vi "Recursive Delete of Registry Key.vi"(8 "error in (no error)":errorcluster, 11 "Path of Key to Delete":string) -> (0 "error out":errorcluster)   [LabVIEW 2011]
uses:
  <vilib>/registry/registry.llb/Registry refnum.ctl
  <vilib>/registry/registry.llb/Registry RtKey.ctl
  <vilib>/registry/registry.llb/Registry SAM.ctl
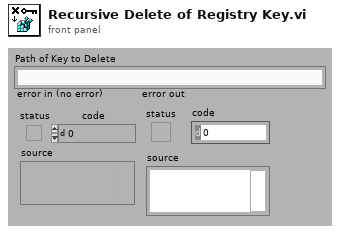
[diagram p1: front panel]
types:
  T1 = typedef "Registry SAM.ctl" = enum32{"KEY_QUERY_VALUE", "KEY_SET_VALUE", "KEY_CREATE_SUB_KEY", "KEY_ENUMERATE_SUB_KEYS", "KEY_NOTIFY", "KEY_CREATE_LINK", "KEY_READ", "KEY_WRITE", "KEY_ALL_ACCESS", "KEY_READ | KEY_WRITE"}
  T2 = typedef "Registry RtKey.ctl" = enum32{"HKEY_CLASSES_ROOT", "HKEY_CURRENT_USER", "HKEY_LOCAL_MACHINE", "HKEY_USERS", "HKEY_PERFORMANCE_DATA", "HKEY_CURRENT_CONFIG", "HKEY_DYN_DATA"}
  T3 = typedef "Registry refnum.ctl" = refnum<k1>
  T4 = cluster{"numSubKeys":i32, "maxSubKeyLen":i32, "maxSubKeyClassLen":i32}
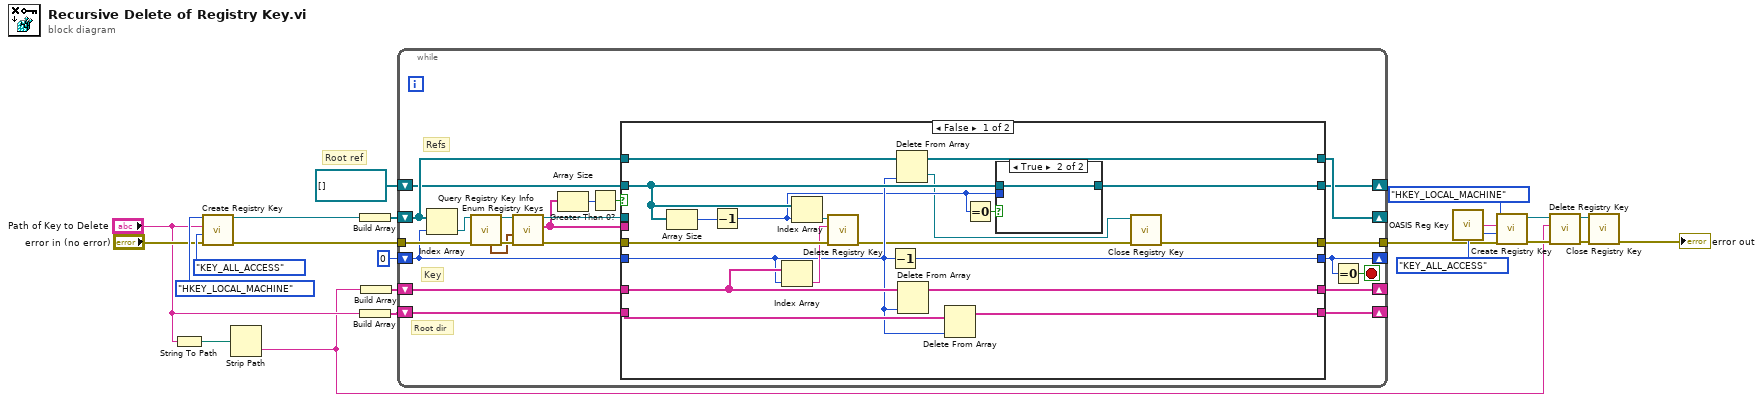
[diagram p0: block diagram]
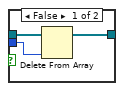
[diagram p2: hidden frame]
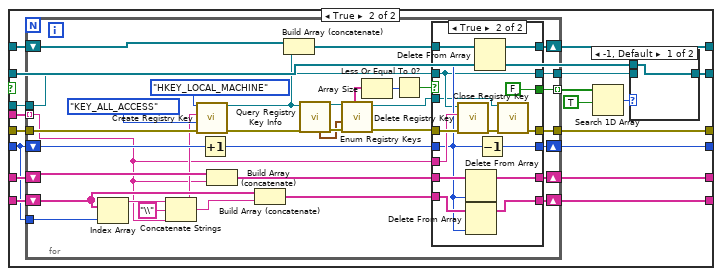
[diagram p3: hidden frame]
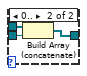
[diagram p4: hidden frame]
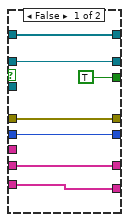
[diagram p5: hidden frame]
diagram:
  # "Root ref"
  n1 = String To Path(string="Path of Key to Delete") -> (path=w3:path)
  n2 = call <vilib>:"Create Registry Key.vi"("error in (no error)"="error in (no error)", "security access mask (KEY_READ | KEY_WRITE)"=Registry_SAM."KEY_ALL_ACCESS", "subkey"="Path of Key to Delete", "root key (HKEY_LOCAL_MACHINE)"=Registry_RtKey."HKEY_LOCAL_MACHINE") -> ("error out"=w5:errorcluster, "refnum out"=w6:T3)  [unwired: 5 in, 1 out]
  n3 = Strip Path(path=w3) -> (name=w1:string)  [unwired: 1 out]
  n4 = Build Array(w6) -> (w19:T3[])
  n5 = Build Array("Path of Key to Delete") -> (w17:string[])
  n6 = Build Array(w1) -> (w18:string[])
  n7 = while {
    tunnel: w5 -> [w40]
    shift-right: [w31] -> _
    shift-left: 0 -> [w34]
    tunnel: [w33] -> w13
    shift-right: [w29] -> _
    shift-left: w19 -> [w30]
    shift-right: [w27] -> _
    shift-left: w18 -> [w28]
    shift-right: [w25] -> _
    shift-left: w17 -> [w26]
    shift-right: [w23] -> _
    shift-left: T3[] [] -> [w24]
    stop <- w44 stop-if-true
    # "Refs"
    # "Root dir"
    # "Key"
    n8 = Index Array(array=w30, index=w34) -> (element=w38:T3)
    n9 = call <vilib>:"Query Registry Key Info.vi"("error in (no error)"=w40, "refnum"=w38) -> ("error out"=w43:errorcluster, "refnum out"=w42:T3, "subkey info"=w41:T4)  [unwired: 5 in, 2 out]
    n10 = call <vilib>:"Enum Registry Keys.vi"("error in (no error)"=w43, "subkey info"=w41, "refnum"=w42) -> ("error out"=w39:errorcluster, "subkeys"=w32:string[], "refnum out"=w37:T3)  [unwired: 6 in]
    n11 = Array Size(array=w32) -> (size(s)=w36:i32)
    n12 = Greater Than 0?(x=w36) -> (x > 0?=w35:bool)
    n13 = case shown="False" w35 {
      tunnel: w39 -> [w63 w84]
      tunnel: w37 -> [_ w74]
      tunnel: w32 -> [_ w80]
      tunnel: w34 -> [w51 w75]
      tunnel: [w50 w85] -> w31
      tunnel: [w46 w83] -> w33
      tunnel: w30 -> [w58 w82]
      tunnel: [w57 w81] -> w29
      tunnel: w28 -> [w56 w78]
      tunnel: [w55 w79] -> w27
      tunnel: w26 -> [w54 w77]
      tunnel: [w53 w76] -> w25
      tunnel: w24 -> [w60 w71]
      tunnel: [w59 w73] -> w23
      frame False {
        n14 = Array Size(array=w60) -> (size(s)=w52:i32)
        n15 = Decrement(x=w52) -> (x-1=w48:i32)
        n16 = Index Array(array=w56, index=w51) -> (element=w62:string)
        n17 = Index Array(array=w60, index=w48) -> (element=w61:T3)
        n18 = call <vilib>:"Delete Registry Key.vi"("error in (no error)"=w63, "subkey"=w62, "refnum"=w61) -> ("error out"=w47:errorcluster)  [unwired: 7 in, 1 out]
        n19 = Decrement(x=w51) -> (x-1=w50:i32)
        n20 = Delete From Array(array=w58, index=w51) -> (deleted portion=w45:T3, array with subset deleted=w57:T3[])  [unwired: 1 in]
        n21 = Delete From Array(array=w56, index=w51) -> (array with subset deleted=w55:string[])  [unwired: 1 in, 1 out]
        n22 = Delete From Array(array=w54, index=w51) -> (array with subset deleted=w53:string[])  [unwired: 1 in, 1 out]
        n23 = Equal To 0?(x=w48) -> (x = 0?=w49:bool)
        n24 = case shown="True" w49 {
          tunnel: w60 -> [w66 w67]
          tunnel: [w65 w67] -> w59
          tunnel: w48 -> [w64 _]
          frame False {
            n25 = Delete From Array(array=w66, index=w64) -> (array with subset deleted=w65:T3[])  [unwired: 1 in, 1 out]
          }
          frame True {
          }
        }
        n26 = call <vilib>:"Close Registry Key.vi"("error in (no error)"=w47, "refnum"=w45) -> ("error out"=w46:errorcluster)  [unwired: 5 in]
      }
      frame True {
        n27 = for {
          tunnel: w84 -> [w121]
          tunnel: [w111] -> w83
          tunnel: w80 -> [w109] mode=indexing
          shift-right: [w110] -> w85
          shift-left: w75 -> [w117]
          shift-right: [w98] -> w81
          shift-left: w82 -> [w119]
          shift-right: [w95] -> w79
          shift-left: w78 -> [w118]
          shift-right: [w94] -> w76
          shift-left: w77 -> [w115]
          tunnel: w75 -> [w114]
          tunnel: w74 -> [w93]
          tunnel: [w92] -> w72
          tunnel: [w91] -> w70 mode=indexing
          n28 = Index Array(array=w115, index=w114) -> (element=w116:string)
          n29 = Concatenate Strings(w116, "\\" ("string"), w109) -> (w113:string)
          n30 = call <vilib>:"Create Registry Key.vi"("error in (no error)"=w121, "security access mask (KEY_READ | KEY_WRITE)"=Registry_SAM."KEY_ALL_ACCESS", "subkey"=w113, "root key (HKEY_LOCAL_MACHINE)"=Registry_RtKey."HKEY_LOCAL_MACHINE") -> ("error out"=w104:errorcluster, "refnum out"=w100:T3)  [unwired: 5 in, 1 out]
          n31 = Increment(x=w117) -> (x+1=w112:i32)
          n32 = Build Array (concatenate)(w118, w109) -> (w96:string[])
          n33 = Build Array (concatenate)(w115, w113) -> (w97:string[])
          n34 = Build Array (concatenate)(w119, w100) -> (w99:T3[])
          n35 = call <vilib>:"Query Registry Key Info.vi"("error in (no error)"=w104, "refnum"=w100) -> ("error out"=w108:errorcluster, "refnum out"=w107:T3, "subkey info"=w102:T4)  [unwired: 5 in, 2 out]
          n36 = call <vilib>:"Enum Registry Keys.vi"("error in (no error)"=w108, "subkey info"=w102, "refnum"=w107) -> ("error out"=w103:errorcluster, "subkeys"=w105:string[], "refnum out"=w90:T3)  [unwired: 6 in]
          n37 = Array Size(array=w105) -> (size(s)=w106:i32)
          n38 = Less Or Equal To 0?(x=w106) -> (x <= 0?=w101:bool)
          n39 = case shown="True" w101 {
            tunnel: w112 -> [w130 w136]
            tunnel: w103 -> [w129 w145]
            tunnel: [w129 w132] -> w111
            tunnel: [w130 w144] -> w110
            tunnel: w109 -> [_ w143]
            tunnel: w99 -> [w128 w142]
            tunnel: [w128 w141] -> w98
            tunnel: w97 -> [w126 w138]
            tunnel: w96 -> [w127 w140]
            tunnel: [w127 w139] -> w95
            tunnel: [w126 w137] -> w94
            tunnel: w93 -> [w125 w135]
            tunnel: [w125 w135] -> w92
            tunnel: [TRUE FALSE] -> w91
            tunnel: w90 -> [_ w131]
            frame False {
            }
            frame True {
              n40 = call <vilib>:"Delete Registry Key.vi"("error in (no error)"=w145, "subkey"=w143, "refnum"=w135) -> ("error out"=w133:errorcluster)  [unwired: 7 in, 1 out]
              n41 = Delete From Array(array=w140, index=w136) -> (array with subset deleted=w139:string[])  [unwired: 1 in, 1 out]
              n42 = Delete From Array(array=w138, index=w136) -> (array with subset deleted=w137:string[])  [unwired: 1 in, 1 out]
              n43 = Delete From Array(array=w142, index=w136) -> (array with subset deleted=w141:T3[])  [unwired: 1 in, 1 out]
              n44 = Decrement(x=w136) -> (x-1=w144:i32)
              n45 = call <vilib>:"Close Registry Key.vi"("error in (no error)"=w133, "refnum"=w131) -> ("error out"=w132:errorcluster)  [unwired: 5 in]
            }
          }
        }
        n46 = Search 1D Array(1D array=w70, element=TRUE) -> (index of element=w68:i32)  [unwired: 1 in]
        n47 = case shown="-1, Default" w68 {
          tunnel: [w86 w89] -> w73
          tunnel: w72 -> [_ w88]
          tunnel: w71 -> [w86 w87]
          frame -1, Default {
          }
          frame 0.. {
            n48 = Build Array (concatenate)(w87, w88) -> (w89:T3[])
          }
        }
      }
    }
    n49 = Equal To 0?(x=w31) -> (x = 0?=w44:bool)
  }
  n50 = call "OASIS Reg Key.vi"() -> ("OASIS Reg Key"=w16:string)  [unwired: 5 in]
  n51 = call <vilib>:"Create Registry Key.vi"("error in (no error)"=w13, "security access mask (KEY_READ | KEY_WRITE)"=Registry_SAM."KEY_ALL_ACCESS", "subkey"=w16, "root key (HKEY_LOCAL_MACHINE)"=Registry_RtKey."HKEY_LOCAL_MACHINE") -> ("error out"=w12:errorcluster, "refnum out"=w11:T3)  [unwired: 5 in, 1 out]
  n52 = call <vilib>:"Delete Registry Key.vi"("error in (no error)"=w12, "subkey"=w1, "refnum"=w11) -> ("error out"=w10:errorcluster, "refnum out"=w9:T3)  [unwired: 7 in]
  n53 = call <vilib>:"Close Registry Key.vi"("error in (no error)"=w10, "refnum"=w9) -> ("error out"=→"error out":errorcluster)  [unwired: 5 in]
